vi "sv_Chirp Wave.vi"(6 "state in":T2={"frequency [Hz]"=20.0, "phase [rad]"=0.0, "elapsed time [s]"=0.0} {"elapsed time [s]" format="%.6f"; "phase [rad]" format="%.6f"; "frequency [Hz]" format="%.2f"}, 7 "frequency spacing":enum16{"Linear", "Logarithmic"}(ring), 8 "sampling info":cluster{"Fs":dbl, "#s":u32}={"Fs"=51200.0, "#s"=1024} {"Fs" format="%.2p"}, 9 "amplitude":dbl=1.0 format="%.2f", 10 "chirp duration [s]":dbl=-1.0, 11 "frequency range":T1={"start frequency [Hz]"=10.0, "stop frequency [Hz]"=10000.0} {"stop frequency [Hz]" format="%.2f"; "start frequency [Hz]" format="%.2f"}) -> (2 "frequency slope":dbl, 3 "chirp wave":dbl[](array[numeric]), 4 "state out":T2={"frequency [Hz]"=20.0, "phase [rad]"=0.0, "elapsed time [s]"=0.0} {"elapsed time [s]" format="%.6f"; "phase [rad]" format="%.6f"; "frequency [Hz]" format="%.2f"})   [LabVIEW 2017, in "SoundVib_Generation.lvlib"]
doc: "Generates a continuous pink noise waveform."
uses:
  <vilib>/addons/_NISVFA/_Generation/SoundVib_Generation.lvlib
  <vilib>/Analysis/1siggen.llb/Ramp Pattern by Samples.vi
  <vilib>/Analysis/NI_AALBase.lvlib
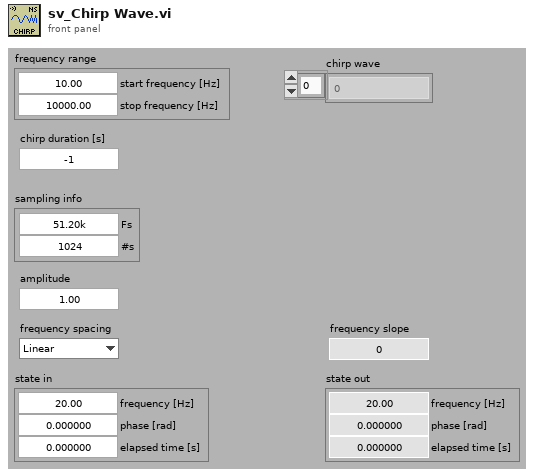
[diagram p1: front panel]
types:
  T1 = cluster{"start frequency [Hz]":dbl, "stop frequency [Hz]":dbl}
  T2 = cluster{"frequency [Hz]":dbl, "phase [rad]":dbl, "elapsed time [s]":dbl}
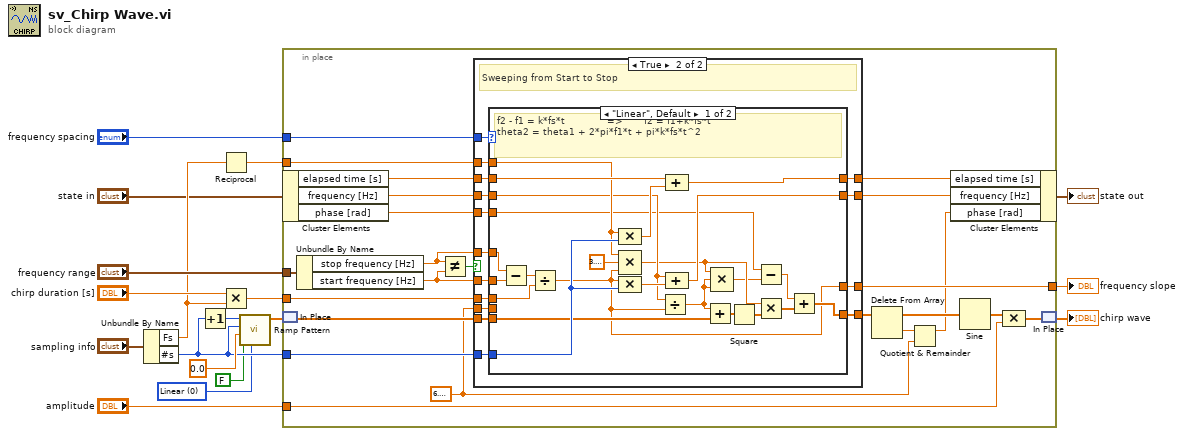
[diagram p0: block diagram]
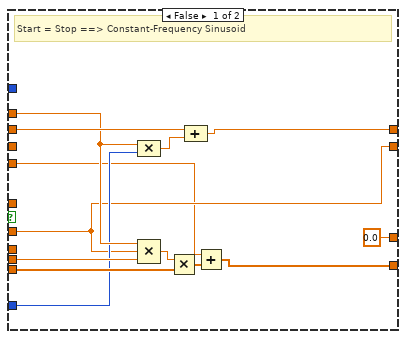
[diagram p2: hidden frame]
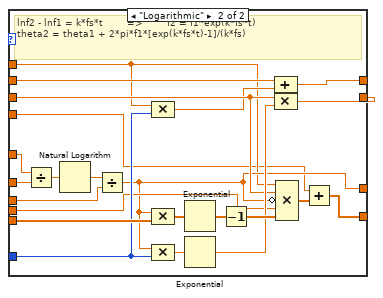
[diagram p3: hidden frame]
diagram:
  w2 = u16 0 items=["Linear", "Logarithmic"] ("type")
  n1 = Unbundle By Name("sampling info") -> ("Fs"=w8:dbl, "#s"=w9:u32)
  n2 = Increment(x=w9) -> (x+1=w11:u32)
  n3 = Reciprocal(x=w8) -> (1/x=w10:dbl)
  n4 = Multiply(x="chirp duration [s]", y=w8) -> (x*y=w7:dbl)
  n5 = call-poly <vilib>:"Ramp Pattern.vi"("type"=w2, "exclude end?"=FALSE, "start"=0.0, "end"=w9, "samples"=w11) -> ("Ramp Pattern"=w4:dbl[])  [unwired: 5 in, 1 out]
  n6 = in-place {
    in-place-border: "amplitude" -> [w41]
    in-place-border: "frequency spacing" -> [w40]
    in-place-border: "frequency range" -> [w39]
    in-place-border: [w25] -> w13
    in-place-border: w10 -> [w37]
    in-place-border: w9 -> [w33]
    in-place-border: w7 -> [w32]
    w24 = 6.283185307179586
    n7 = in-place-cluster #1("state in") -> ("elapsed time [s]"=w31:dbl, "frequency [Hz]"=w30:dbl, "phase [rad]"=w23:dbl)
    n8 = in-place-match #2(w4) -> (w27:dbl[])
    n9 = Unbundle By Name(w39) -> ("stop frequency [Hz]"=w20:dbl, "start frequency [Hz]"=w19:dbl)
    n10 = Not Equal?(x=w20, y=w19) -> (x != y?=w21:bool)
    n11 = case shown="True" w21 {
      tunnel: w40 -> [_ w69]
      tunnel: w37 -> [w50 w68]
      tunnel: [w42 w67] -> w36
      tunnel: w33 -> [w47 w66]
      tunnel: w20 -> [_ w65]
      tunnel: w19 -> [w45 w64]
      tunnel: w32 -> [_ w63]
      tunnel: w31 -> [w53 w62]
      tunnel: w30 -> [_ w61]
      tunnel: [w52 w60] -> w29
      tunnel: [w45 w59] -> w28
      tunnel: w27 -> [w48 w58]
      tunnel: [0.0 w57] -> w25
      tunnel: w24 -> [w49 w56]
      tunnel: w23 -> [w44 w55]
      frame False {
        # "Start = Stop ==> Constant-Frequency Sinusoid"
        n12 = Compound Arithmetic op=MULTIPLY(w50, w47) -> (w54:dbl)
        n13 = Compound Arithmetic op=MULTIPLY(w50, w45, w49) -> (w46:dbl)
        n14 = Multiply(x=w46, y=w48) -> (x*y=w43:dbl[])
        n15 = Compound Arithmetic op=ADD(w53, w54) -> (w52:dbl)
        n16 = Add(x=w44, y=w43) -> (x+y=w42:dbl[])
      }
      frame True {
        # "Sweeping from Start to Stop"
        n17 = case shown="\"Linear\", Default" w69 {
          tunnel: w61 -> [w85 w109]
          tunnel: w55 -> [w81 w94]
          tunnel: w58 -> [w84 w114]
          tunnel: w66 -> [w91 w108]
          tunnel: w68 -> [w86 w95]
          tunnel: w62 -> [w89 w106]
          tunnel: [w88 w105] -> w60
          tunnel: [w87 w104] -> w59
          tunnel: [w75 w103] -> w67
          tunnel: [w70 w96] -> w57
          tunnel: w65 -> [w73 w100]
          tunnel: w64 -> [w72 w99]
          tunnel: w63 -> [w71 w98]
          tunnel: w56 -> [_ w97]
          frame "Linear", Default {
            # "f2 - f1 = k*fs*t              =>       f2 = f1+k*fs*t\ntheta2 = theta1 + 2*pi*f1*t + pi*k*fs*t^2"
            n18 = Subtract(x=w73, y=w72) -> (x-y=w74:dbl)
            n19 = Divide(x=w74, y=w71) -> (x/y=w70:dbl)
            n20 = Compound Arithmetic op=MULTIPLY(w86, w91) -> (w90:dbl)
            n21 = Compound Arithmetic op=MULTIPLY(w86, 3.141592653589793, w70) -> (w79:dbl)
            n22 = Compound Arithmetic op=MULTIPLY(w70, w91) -> (w93:dbl)
            n23 = Divide(x=w85, y=w70) -> (x/y=w80:dbl)
            n24 = Compound Arithmetic op=ADD(w89, w90) -> (w88:dbl)
            n25 = Compound Arithmetic op=ADD(w85, w93) -> (w87:dbl)
            n26 = Add(x=w80, y=w84) -> (x+y=w83:dbl[])
            n27 = Compound Arithmetic op=MULTIPLY(w79, w80, w80) -> (w78:dbl)
            n28 = Square(x=w83) -> (x^2=w82:dbl[])
            n29 = Subtract(x=w81, y=w78) -> (x-y=w77:dbl)
            n30 = Multiply(x=w79, y=w82) -> (x*y=w76:dbl[])
            n31 = Add(x=w77, y=w76) -> (x+y=w75:dbl[])
          }
          frame "Logarithmic" {
            # "lnf2 - lnf1 = k*fs*t        =>        f2 = f1*exp(k*fs*t)\ntheta2 = theta1 + 2*pi*f1*[exp(k*fs*t)-1]/(k*fs)"
            n32 = Divide(x=w100, y=w99) -> (x/y=w101:dbl)
            n33 = Natural Logarithm(1:w101) -> (0:w102:dbl)
            n34 = Divide(x=w102, y=w98) -> (x/y=w96:dbl)
            n35 = Compound Arithmetic op=MULTIPLY(w95, w108) -> (w107:dbl)
            n36 = Compound Arithmetic op=MULTIPLY(w96, w114) -> (w116:dbl[])
            n37 = Compound Arithmetic op=MULTIPLY(w96, w108) -> (w112:dbl)
            n38 = Exponential(1:w116) -> (0:w113:dbl[])
            n39 = Exponential(1:w112) -> (0:w110:dbl)
            n40 = Decrement(x=w113) -> (x-1=w111:dbl[])
            n41 = Compound Arithmetic op=ADD(w106, w107) -> (w105:dbl)
            n42 = Compound Arithmetic op=MULTIPLY(w109, w110) -> (w104:dbl)
            n43 = Compound Arithmetic op=MULTIPLY(w95, w109, invert w96, w97, w111) -> (w115:dbl[])
            n44 = Add(x=w94, y=w115) -> (x+y=w103:dbl[])
          }
        }
      }
    }
    n45 = Delete From Array(array=w36) -> (deleted portion=w34:dbl, array with subset deleted=w35:dbl[])  [unwired: 2 in]
    n46 = Quotient & Remainder(x=w34, y=w24) -> (x-y*floor(x/y)=w22:dbl)  [unwired: 1 out]
    n47 = in-place-cluster #1("elapsed time [s]"=w29, "frequency [Hz]"=w28, "phase [rad]"=w22) -> (→"state out":T2)
    n48 = Sine(x=w35) -> (sin(x)=w38:dbl[])
    n49 = Compound Arithmetic op=MULTIPLY(w38, w41) -> (w26:dbl[])
    n50 = in-place-match #2(w26) -> (→"chirp wave":dbl[])
  }
  "frequency slope" <- w13
